vi "火焰参数.vi"(7 "像素当量单位":string, 8 "?":string, 9 "?":string, 10 "Image 2":T2, 11 "Image":T2) -> ()   [LabVIEW 2018]
uses:
  <vilib>/vision/Image Controls.llb/IMAQ Image.ctl
  <vilib>/vision/NI_Vision_Development_Module.lvlib
panel:
  out "?":string
  in  "参数单位":bool
  out "?":T1
  out "?":string
  in  "查看第几部分叠加火焰":i32=1
  in  "取消查看":bool
  in  "查看第几部分单帧火焰":i32=1
  out "?":string
  out "?":T1
  # "火焰分割参数"
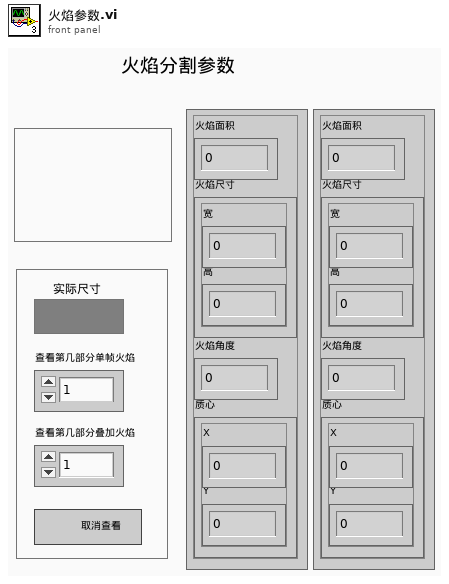
[diagram p1: front panel]
types:
  T1 = cluster{"火焰面积":dbl, "火焰尺寸":cluster{"宽":dbl, "高":dbl}, "火焰角度":dbl, "质心":cluster{"X":dbl, "Y":dbl}}
  T2 = typedef "IMAQ Image.ctl" = refnum<image>
  T3 = cluster{"Area":dbl, "Number of Holes":dbl, "Bounding Rect":cluster{"Left":dbl, "Top":dbl, "Right":dbl, "Bottom":dbl}, "Center of Mass":cluster{"X":dbl, "Y":dbl}, "Orientation":dbl, "Dimensions":cluster{"Width":dbl, "Height":dbl}}[]
  T4 = cluster{"Area":dbl, "Number of Holes":dbl, "Bounding Rect":cluster{"Left":dbl, "Top":dbl, "Right":dbl, "Bottom":dbl}, "Center of Mass":cluster{"X":dbl, "Y":dbl}, "Orientation":dbl, "Dimensions":cluster{"Width":dbl, "Height":dbl}}
  T5 = cluster{dbl, "Dimensions":cluster{"Width":dbl, "Height":dbl}, "Orientation":dbl, "Center of Mass":cluster{"X":dbl, "Y":dbl}}
  T6 = cluster{"Area":dbl, "Dimensions":cluster{"Width":dbl, "Height":dbl}, "Orientation":dbl, "Center of Mass":cluster{"X":dbl, "Y":dbl}}
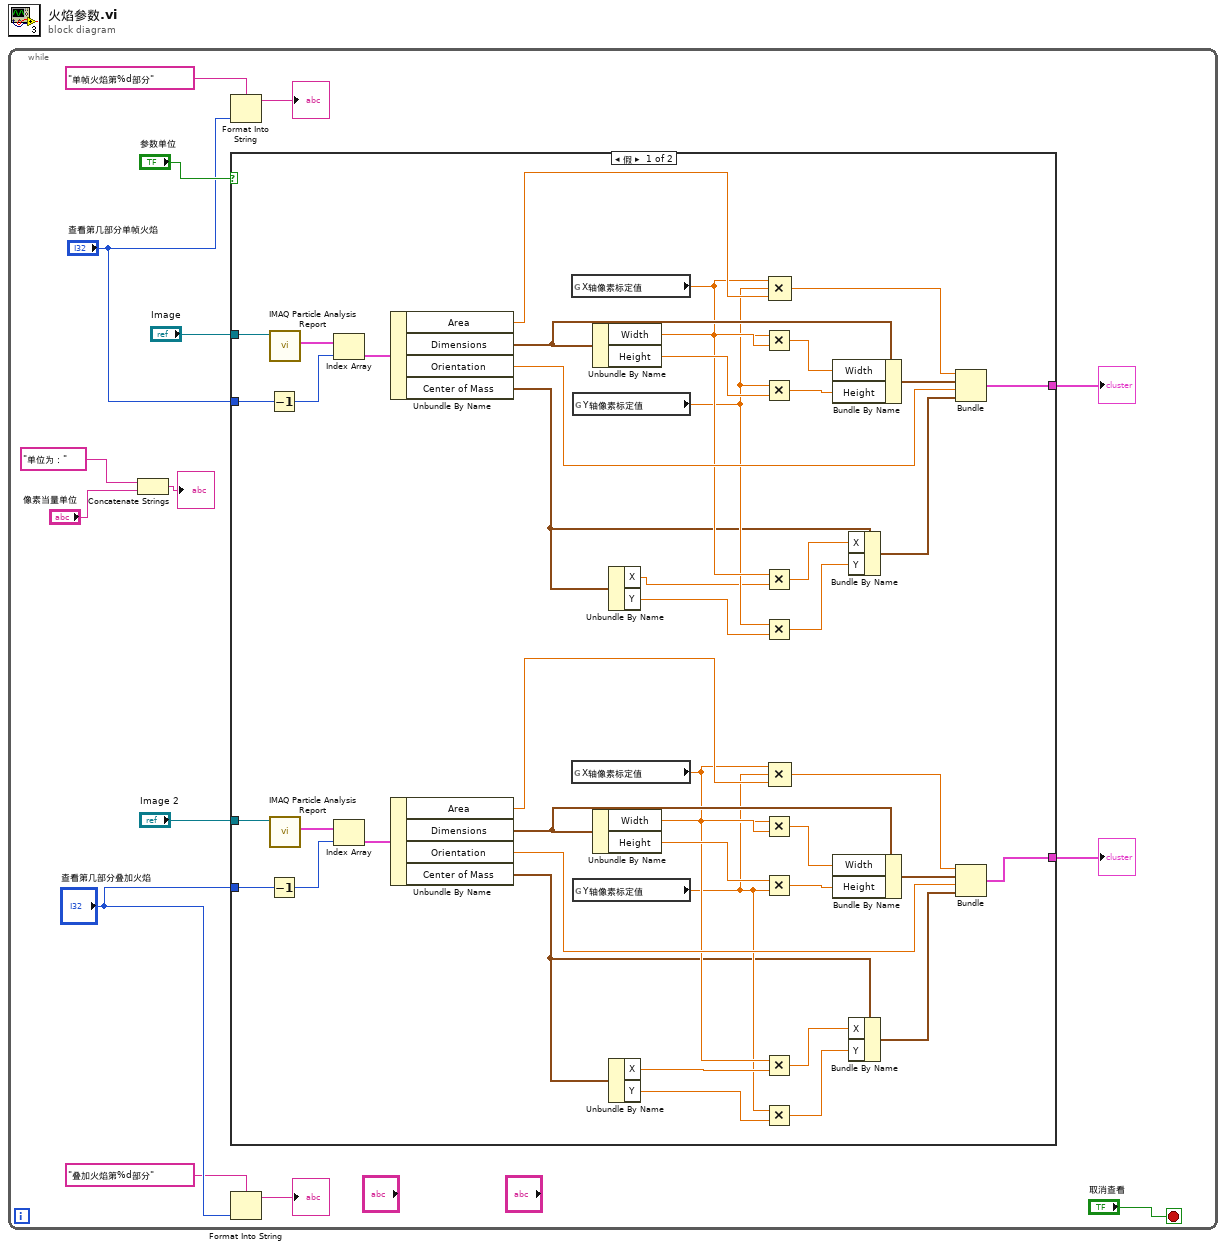
[diagram p0: block diagram]
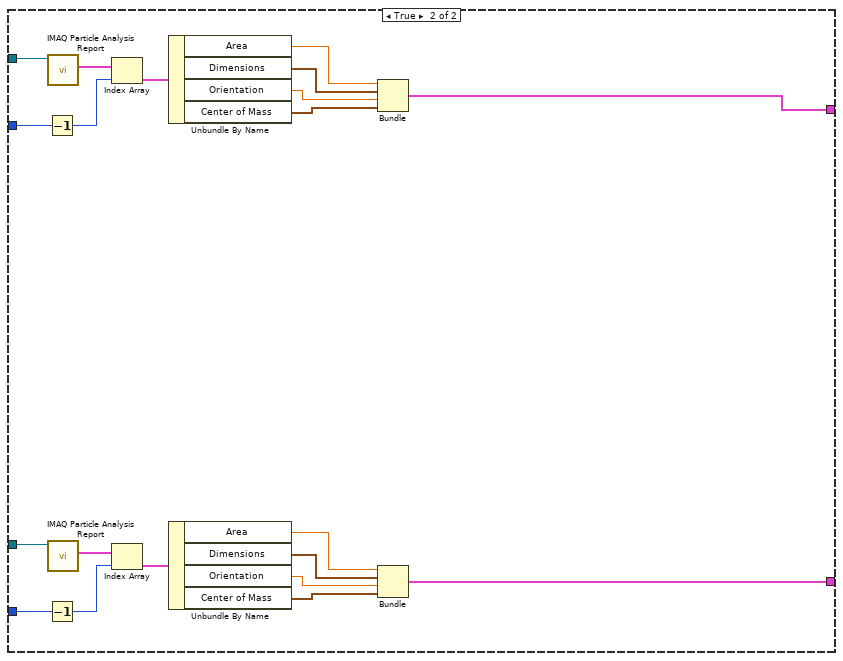
[diagram p2: hidden frame]
diagram:
  n1 = while {
    stop <- "取消查看" stop-if-true
    n2 = Concatenate Strings("单位为：", "像素当量单位") -> (→"?":string)
    n3 = Format Into String(format string="单帧火焰第%d部分" ("初始字符串"), "查看第几部分单帧火焰") -> (resulting string=→"?":string)  [unwired: 2 in, 1 out]
    n4 = case shown="假" "参数单位" {
      tunnel: "Image" -> [w59 w81]
      tunnel: "查看第几部分单帧火焰" -> [w56 w79]
      tunnel: "查看第几部分叠加火焰" -> [w57 w76]
      tunnel: "Image 2" -> [w58 w74]
      tunnel: [w51 w62] -> w5
      tunnel: [w47 w63] -> w4
      frame False {
        n5 = Decrement(x=w56) -> (x-1=w61:i32)
        n6 = Decrement(x=w57) -> (x-1=w60:i32)
        n7 = call "IMAQ Particle Analysis Report"("Image"=w59) -> ("Particle Reports (Pixels)"=w50:T3)  [unwired: 5 in, 5 out]
        n8 = call "IMAQ Particle Analysis Report"("Image"=w58) -> ("Particle Reports (Pixels)"=w49:T3)  [unwired: 5 in, 5 out]
        n9 = Index Array(array=w50, index=w61) -> (element=w54:T4)
        n10 = Index Array(array=w49, index=w60) -> (element=w52:T4)
        n11 = Unbundle By Name(w54) -> ("Area"=w48:dbl, "Dimensions"=w28:cluster{"Width":dbl, "Height":dbl}, "Orientation"=w55:dbl, "Center of Mass"=w16:cluster{"X":dbl, "Y":dbl})
        n12 = Unbundle By Name(w52) -> ("Area"=w45:dbl, "Dimensions"=w43:cluster{"Width":dbl, "Height":dbl}, "Orientation"=w53:dbl, "Center of Mass"=w33:cluster{"X":dbl, "Y":dbl})
        n13 = global read "全局变量.vi" "X轴像素标定值"() -> (w23:dbl)
        n14 = global read "全局变量.vi" "X轴像素标定值"() -> (w37:dbl)
        n15 = global read "全局变量.vi" "Y轴像素标定值"() -> (w22:dbl)
        n16 = global read "全局变量.vi" "Y轴像素标定值"() -> (w35:dbl)
        n17 = Unbundle By Name(w28) -> ("Width"=w29:dbl, "Height"=w25:dbl)
        n18 = Unbundle By Name(w43) -> ("Width"=w42:dbl, "Height"=w40:dbl)
        n19 = Unbundle By Name(w16) -> ("X"=w21:dbl, "Y"=w20:dbl)
        n20 = Unbundle By Name(w33) -> ("X"=w36:dbl, "Y"=w34:dbl)
        n21 = Multiply(x=w23, y=w29) -> (x*y=w27:dbl)
        n22 = Multiply(x=w22, y=w25) -> (x*y=w26:dbl)
        n23 = Multiply(x=w23, y=w21) -> (x*y=w19:dbl)
        n24 = Multiply(x=w22, y=w20) -> (x*y=w18:dbl)
        n25 = Multiply(x=w37, y=w42) -> (x*y=w41:dbl)
        n26 = Multiply(x=w40, y=w35) -> (x*y=w39:dbl)
        n27 = Multiply(x=w37, y=w36) -> (x*y=w32:dbl)
        n28 = Multiply(x=w35, y=w34) -> (x*y=w31:dbl)
        n29 = Compound Arithmetic op=MULTIPLY(w23, w22, w48) -> (w46:dbl)
        n30 = Compound Arithmetic op=MULTIPLY(w37, w35, w45) -> (w44:dbl)
        n31 = Bundle By Name(cluster=w28, "Width"=w27, "Height"=w26) -> (w24:cluster{"Width":dbl, "Height":dbl})
        n32 = Bundle By Name(cluster=w43, "Width"=w41, "Height"=w39) -> (w38:cluster{"Width":dbl, "Height":dbl})
        n33 = Bundle By Name(cluster=w16, "X"=w19, "Y"=w18) -> (w17:cluster{"X":dbl, "Y":dbl})
        n34 = Bundle By Name(cluster=w33, "X"=w32, "Y"=w31) -> (w30:cluster{"X":dbl, "Y":dbl})
        n35 = Bundle(w46, "Dimensions"=w24, "Orientation"=w55, "Center of Mass"=w17) -> (w47:T5)  [unwired: 1 in]
        n36 = Bundle(w44, "Dimensions"=w38, "Orientation"=w53, "Center of Mass"=w30) -> (w51:T5)  [unwired: 1 in]
      }
      frame True {
        n37 = Decrement(x=w79) -> (x-1=w78:i32)
        n38 = Decrement(x=w76) -> (x-1=w77:i32)
        n39 = call "IMAQ Particle Analysis Report"("Image"=w81) -> ("Particle Reports (Pixels)"=w80:T3)  [unwired: 5 in, 5 out]
        n40 = call "IMAQ Particle Analysis Report"("Image"=w74) -> ("Particle Reports (Pixels)"=w75:T3)  [unwired: 5 in, 5 out]
        n41 = Index Array(array=w80, index=w78) -> (element=w64:T4)
        n42 = Index Array(array=w75, index=w77) -> (element=w65:T4)
        n43 = Unbundle By Name(w64) -> ("Area"=w73:dbl, "Dimensions"=w72:cluster{"Width":dbl, "Height":dbl}, "Orientation"=w71:dbl, "Center of Mass"=w70:cluster{"X":dbl, "Y":dbl})
        n44 = Unbundle By Name(w65) -> ("Area"=w66:dbl, "Dimensions"=w67:cluster{"Width":dbl, "Height":dbl}, "Orientation"=w68:dbl, "Center of Mass"=w69:cluster{"X":dbl, "Y":dbl})
        n45 = Bundle("Area"=w73, "Dimensions"=w72, "Orientation"=w71, "Center of Mass"=w70) -> (w63:T6)  [unwired: 1 in]
        n46 = Bundle("Area"=w66, "Dimensions"=w67, "Orientation"=w68, "Center of Mass"=w69) -> (w62:T6)  [unwired: 1 in]
      }
    }
    "?" <- w5
    "?" <- w4
    n47 = Format Into String(format string="叠加火焰第%d部分" ("初始字符串"), "查看第几部分叠加火焰") -> (resulting string=→"?":string)  [unwired: 2 in, 1 out]
  }
